vi "S2C_ExeDeferUpdates.vi"(8 "Error In":errorcluster, 11 "Defer?":bool) -> (0 "Error Out":errorcluster)   [LabVIEW 2015]
uses:
  Globals/S2C_Globals.vi
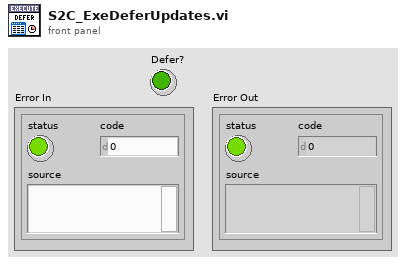
[diagram p1: front panel]
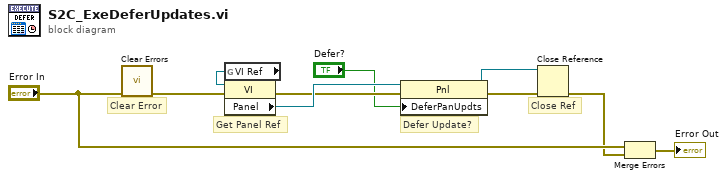
[diagram p0: block diagram]
diagram:
  # "Clear Error"
  # "Close Ref"
  # "Defer Update?"
  # "Get Panel Ref"
  n1 = call <vilib>:"Clear Errors.vi"("error in (no error)"="Error In") -> ("error out"=w4:errorcluster)  [unwired: 5 in, 1 out]
  n2 = global read "S2C_Globals.vi" "VI Ref"() -> (w10:refnum<vi>)
  n3 = property class="VI"(reference=w10, error in=w4) -> (error out=w8:errorcluster, "Panel"=w9:refnum<vi>)  [unwired: 1 out]
  n4 = property class="Pnl"(reference=w9, error in=w8, "DeferPanUpdts"="Defer?") -> (reference out=w5:refnum<vi>, error out=w6:errorcluster)
  n5 = Close Reference(reference=w5, error in (no error)=w6) -> (error out=w2:errorcluster)
  n6 = Merge Errors("Error In", w2) -> (→"Error Out":errorcluster)
